vi "APD-counter-synchronized.vi"(0 "ao_to_write":tag="Dev1/ao1", 4 "APD_signal":tag="/Dev1/PFI8", 5 "error in (no error)":errorcluster, 6 "y_start_um":dbl=4.0 format="%.3f", 8 "y_end_um":dbl=6.0 format="%.3f", 10 "Duration_s":dbl=1.0 format="%#_6p", 12 "DAQ sampling rate":dbl=10000.0 format="%#_6p") -> (14 "time tags":u32[](array[numeric])=[1617, 8514, 12274, 20565, 34917, 35402, 37265, 38238, 57954, 68377, 79767, 93435, 95330, 115161, 119575, 126232, 134280, 173482, 175010, 177269, 185202, 187516, 187525, 187814, 188411, 189607, 197427, 217503, 223614, 233596, 240824, 256808, 266059, 270070, 271549, 273666, 274381, 279664, 282850, 287407, 293024, 300860, 320469, 331194, 388082, 391502, 397052, 412341, 413800, 451549, 454051, 488548, 547543, 551076, 552583, 586653, 599650, 613877, 615921, 642961, 646267, 647470, 648566, 683015, 686993, 694317, 710159, 710543, 751020, 763526, 767844, 771220, 794182, 809071, 812953, 822705, 850006, 865624, 875877, 879061, 895901, 900981, 902825, 903577, 906993, 907554, 914434, 916405, 921246, 923738, 936250, 936601, 939722, 948191, 976061, 977403, 979255, 988197, 1004150, 1011377, 1023293, 1025748, 1033762, 1036676, 1037210, 1077098, 1094656, 1098932, 1113325, 1123736, 1123910, 1134400, 1136024, 1143608, 1170409, 1213828, 1232961, 1237449, 1259376, 1267857, 1274171, 1282019, 1286854, 1310462, 1313126, 1315046, 1324275, 1326810, 1332178, 1340368, 1340407, 1343990, 1345221, 1346964, 1364694, 1388750, 1391710, 1403678, 1408248, 1428588, 1444290, 1445629, 1449529, 1452777, 1456715, 1467693, 1479877, 1481248, 1486037, 1497559, 1498462, 1506000, 1507373, 1508422, 1509540, 1510507, 1512549, 1517522, 1522108, 1529163, 1558683, 1564453, 1578897, 1584884, 1589263, 1622523, 1639047, 1640280, 1653969, 1667907, 1686341, 1692400, 1702828, 1706400, 1709526, 1713264, 1716614, 1718721, 1721994, 1735244, 1736688, 1739237, 1762850, 1778098, 1784274, 1786663, 1790948, 1805134, 1810522, 1814629, 1836014, 1840078, 1842022, 1861394, 1878208, 1894207, 1919233, 1923567, 1933515, 1951072, 1951153, 1955923, 1967743, 1970393, 1973969, 1977369, 1978257, 1986658, 1990762, 2017254, 2018231, 2022980, 2036748, 2051136, 2068002, 2077318, 2092650, 2101140, 2112303, 2132887, 2134211, 2164113, 2171564, 2173231, 2188929, 2192828, 2195583, 2196607, 2219129, 2224786, 2229299, 2240229, 2240568, 2248558, 2278572, 2298996, 2305229, 2308700, 2313991, 2345345, 2346179, 2349865, 2350771, 2382508, 2389153, 2390999, 2408371, 2428081, 2433877, 2433926, 2435328, 2437892, 2454139, 2457236, 2475748, 2480449, 2483319, 2492985, 2501361, 2526711, 2532104, 2537449, 2540493, 2545042, 2548591, 2560696, 2566230, 2570890, 2580490, 2600440, 2609949, 2610561, 2611858, 2612448, 2615675, 2635002, 2640843, 2643937, 2658169, 2703087, 2707384, 2712186, 2725379, 2773349, 2775106, 2784948, 2785927, 2786930, 2792713, 2796971, 2814031, 2822352, 2835497, 2835845, 2838919, 2840082, 2841672, 2859967, 2872433, 2879793, 2882072, 2889857, 2897761, 2907259, 2929097, 2963378, 2981447, 2989320, 3002384, 3002385, 3003328, 3011854, 3020261, 3021488, 3029005, 3030028, 3035148, 3059511, 3063096, 3069096, 3077896, 3081773, 3099736, 3146787, 3151070, 3153237, 3159851, 3169791, 3184967, 3190957, 3199514, 3202886, 3205088, 3209452, 3228110, 3235052, 3239233, 3246402, 3247518, 3258710, 3259514, 3276763, 3288042, 3321055, 3321903, 3326046, 3355279, 3358734, 3399824, 3406786, 3423548, 3430377, 3430834, 3432472, 3455758, 3456988, 3465084, 3471831, 3475563, 3497296, 3498536, 3506930, 3509738, 3509998, 3538736, 3538762, 3555497, 3566294, 3571416, 3574354, 3587298, 3594158, 3596294, 3597984, 3609878, 3610183, 3619254, 3623133, 3629713, 3635571, 3641115, 3663964, 3670086, 3679821, 3695717, 3697137, 3706852, 3715146, 3728389, 3766001, 3780817, 3802848, 3808019, 3818393, 3830970, 3843232, 3845469, 3864680, 3872910, 3880489, 3882867, 3896587, 3902984, 3919045, 3927836, 3948484, 3952876, 3958522, 3960194, 3972452, 3977978, 4015413, 4026230, 4031811, 4033763, 4037156, 4073209, 4078826, 4078964, 4088360, 4091171, 4096204, 4103351, 4105273, 4126221, 4130227, 4131168, 4164045, 4166878, 4178284, 4210808, 4214700, 4225379, 4235697, 4239456, 4239652, 4243811, 4244908, 4245750, 4259680, 4266654, 4267090, 4269674, 4277689, 4279478, 4288143, 4289477, 4289528, 4316961, 4318563, 4328159, 4344085, 4350067, 4354935, 4357706, 4365546, 4367346, 4383457, 4388029, 4420363, 4435182, 4436109, 4438820, 4468514, 4478175, 4491660, 4492390, 4497102, 4501457, 4501586, 4512174, 4517070, 4518450, 4536838, 4547886, 4555313, 4556110, 4571596, 4591440, 4602493, 4606762, 4617052, 4644899, 4647553, 4657592, 4672401, 4680982, 4693672, 4696454, 4721246, 4746514, 4748546, 4787883, 4798872, 4811344, 4818805, 4821017, 4828436, 4828492, 4828736, 4841201, 4842107, 4859124, 4865880, 4868886, 4872581, 4879021, 4894944, 4917909, 4922087, 4928487, 4928645, 4964638, 4966510, 4973708, 4983803, 4988440, 4994500, 4998320, 5005289, 5035839, 5039124, 5041040, 5048608, 5052074, 5056335, 5060012, 5074947, 5089912, 5111388, 5118788, 5129501, 5130484, 5156063, 5161939, 5173418, 5176262, 5177784, 5180116, 5217588, 5224915, 5258746, 5268307, 5275408, 5297246, 5309159, 5321253, 5328915, 5330134, 5344478, 5349137, 5365467, 5385955, 5398314, 5404550, 5422605, 5423964, 5431856, 5439427, 5444547, 5459606, 5464748, 5473439, 5480165, 5482909, 5484531, 5508669, 5517179, 5536432, 5552946, 5553034, 5560309, 5565589, 5578409, 5579291, 5596776, 5602314, 5605526, 5612381, 5612652, 5622551, 5629364, 5633164, 5637568, 5647785, 5662593, 5663027, 5678087, 5683696, 5707814, 5708040, 5727142, 5739286, 5743393, 5764846, 5767510, 5778919, 5785074, 5788885, 5790436, 5792182, 5794935, 5815798, 5822258, 5847673, 5849629, 5849702, 5852683, 5853644, 5859227, 5864019, 5866082, 5867143, 5888339, 5896516, 5903365, 5919809, 5927912, 5930228, 5932718, 5936422, 5940913, 5942272, 5953828, 5960268, 5966370, 5967906, 5993952, 5994649, 6000191, 6001891, 6035036, 6038421, 6041090, 6050830, 6052556, 6053826, 6056856, 6057097, 6080835, 6088757, 6091135, 6099057, 6102434, 6114932, 6116858, 6129607, 6141016, 6143043, 6152242, 6156105, 6157624, 6159513, 6161373, 6163582, 6178386, 6187956, 6188493, 6205026, 6233167, 6249963, 6263153, 6264365, 6267125, 6267997, 6270213, 6276638, 6281128, 6286842, 6297236, 6302123, 6307585, 6308029, 6327542, 6344909, 6359615, 6368399, 6369002, 6370874, 6424638, 6439503, 6446102, 6461496, 6463502, 6480104, 6494766, 6496031, 6508645, 6519056, 6523380, 6528804, 6554973, 6556902, 6569896, 6571252, 6581020, 6583224, 6584923, 6599291, 6606595, 6614440, 6624564, 6628476, 6632318, 6637716, 6638169, 6644791, 6650232, 6651619, 6656068, 6667291, 6667510, 6704324, 6706226, 6711263, 6719627, 6724016, 6727619, 6756251, 6765545, 6781244, 6785334, 6798675, 6809716, 6817328, 6820211, 6856900, 6868094, 6899041, 6904923, 6909615, 6919040, 6923653, 6936054, 6939203, 6948855, 6953704, 6956189, 6961686, 6973803, 6976824, 6984715, 7001385, 7014029, 7018130, 7019144, 7023351, 7028702, 7033179, 7039934, 7074129, 7076269, 7077132, 7095149, 7099400, 7104359, 7110045, 7115025, 7126495, 7135263, 7158151, 7162036, 7187178, 7189383, 7194225, 7208639, 7208746, 7213943, 7282317, 7299353, 7301721, 7314437, 7316458, 7326789, 7334609, 7337898, 7339472, 7344845, 7346255, 7349370, 7356432, 7366135, 7374208, 7376719, 7380782, 7388813, 7388943, 7397243, 7401920, 7408246, 7416961, 7434816, 7435896, 7439219, 7454399, 7455070, 7459639, 7474225, 7490642, 7491990, 7502524, 7506416, 7511657, 7511671, 7514649, 7519099, 7530651, 7536651, 7549344, 7562326, 7563224, 7564770, 7569785, 7577790, 7583357, 7586769, 7589907, 7592271, 7602685, 7615016, 7621713, 7627357, 7659690, 7661778, 7669294, 7669581, 7681622, 7705966, 7711336, 7713905, 7715976, 7725547, 7737879, 7748149, 7754644, 7757162, 7758005, 7760640, 7774067, 7782750, 7800584, 7806004, 7807595, 7810954, 7812385, 7831951, 7844263, 7852555, 7859270, 7875341, 7891990, 7893385, 7909423, 7917565, 7922227, 7970722, 7973979, 7976651, 7986173, 7988731, 7996540, 7997442, 8002024, 8005784, 8008548, 8015237, 8016979, 8018636, 8031638, 8036817, 8051972, 8052911, 8061175, 8063984, 8071339, 8075799, 8080806, 8082777, 8092643, 8095235, 8101005, 8103243, 8103501, 8105684, 8108064, 8118580, 8130143, 8131594, 8139319, 8142296, 8147224, 8150515, 8157836, 8162474, 8167935, 8169793, 8173237, 8174026, 8174599, 8190819, 8198129, 8216513, 8218408, 8227556, 8230675, 8232058, 8232376, 8237816, 8252618, 8264563, 8276111, 8287066, 8309355, 8310996, 8316353, 8330239, 8332140, 8346844, 8354814, 8379426, 8400413, 8415506, 8417231, 8429309, 8429562, 8448711, 8453931, 8465139, 8468917, 8476213, 8491690, 8507968, 8512199, 8521587, 8525347, 8530588, 8532568, 8533136, 8533606, 8535767, 8542964, 8551744, 8557349, 8568057, 8579623, 8591329, 8630869, 8631263, 8641524, 8641540, 8645573, 8657240, 8659153, 8661211, 8670372, 8671613, 8688464, 8700013, 8705979, 8711129, 8716432, 8727138, 8732652, 8754294, 8760296, 8773752, 8775389, 8792686, 8798218, 8806915, 8806957, 8808256, 8808423, 8810238, 8811551, 8815337, 8815338, 8823424, 8824807, 8831585, 8833635, 8842125, 8849130, 8855007, 8861026, 8862986, 8867363, 8882422, 8902876, 8905207, 8906718, 8911015, 8930178, 8932604, 8943618, 8954223, 8958968, 8959609, 8980355, 8980858, 8985305, 8998408, 9009003, 9036042, 9040401, 9044806, 9047366, 9052151, 9067578, 9068225, 9127447, 9145363, 9146347, 9149805, 9157603, 9162213, 9166615, 9170985, 9184377, 9192907, 9198452, 9201877, 9204403, 9212852, 9214432, 9223940, 9224233, 9228419, 9232814, 9238431, 9239957, 9249919, 9255933, 9262012, 9268098, 9279058, 9279456, 9287255, 9295881, 9296488, 9304065, 9316119, 9343190, 9357714, 9364199, 9365191, 9369210, 9378347, 9387386, 9405033, 9435254, 9437668, 9437972, 9438398, 9440121, 9440983, 9449780, 9455423, 9456955, 9463983, 9495248, 9504104, 9554094, 9573156, 9580807, 9582784, 9591248, 9592954, 9597285, 9605408, 9605979, 9606407, 9616770, 9632422, 9635038, 9647403, 9684806, 9696212, 9722896, 9725217, 9729213, 9740910, 9752284, 9774418, 9786059, 9787440, 9788436, 9795933, 9804987, 9809372, 9812795, 9822094, 9827265, 9833549, 9837013, 9837305, 9840632, 9840891, 9849124, 9856510, 9870947, 9890659, 9892186, 9898537, 9912117, 9914470, 9921183, 9942452, 9948337, 9957854, 9959132, 9964622, 9976656, 9987644, 9999037, 10001684, 10004443, 10025300], 15 "counts":i32=1118, 16 "clock cycles":i32=10000000, 19 "error out":errorcluster)   [LabVIEW 2018]
uses:
  <vilib>/Analysis/1siggen.llb/Ramp Pattern by Samples.vi
  GLOBAL_VAR.vi
  <vilib>/Analysis/NI_AALBase.lvlib
panel:
  out "signal_to_write":waveform(dbl)(graph)={"t0"=timestamp(0 s since 1904-01-01), "dt"=0.0001, "Y"=array[10000 elements]}
  out "#daq samples":i32=10000
  # "Analog Output is a linear ramp"
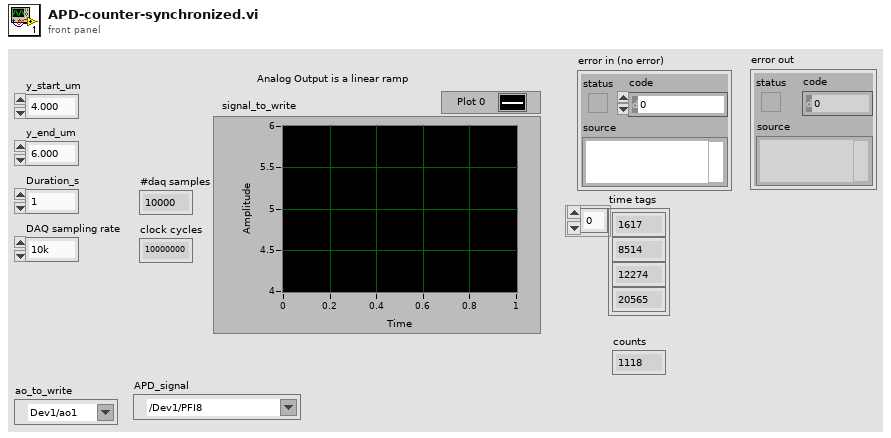
[diagram p1: front panel]
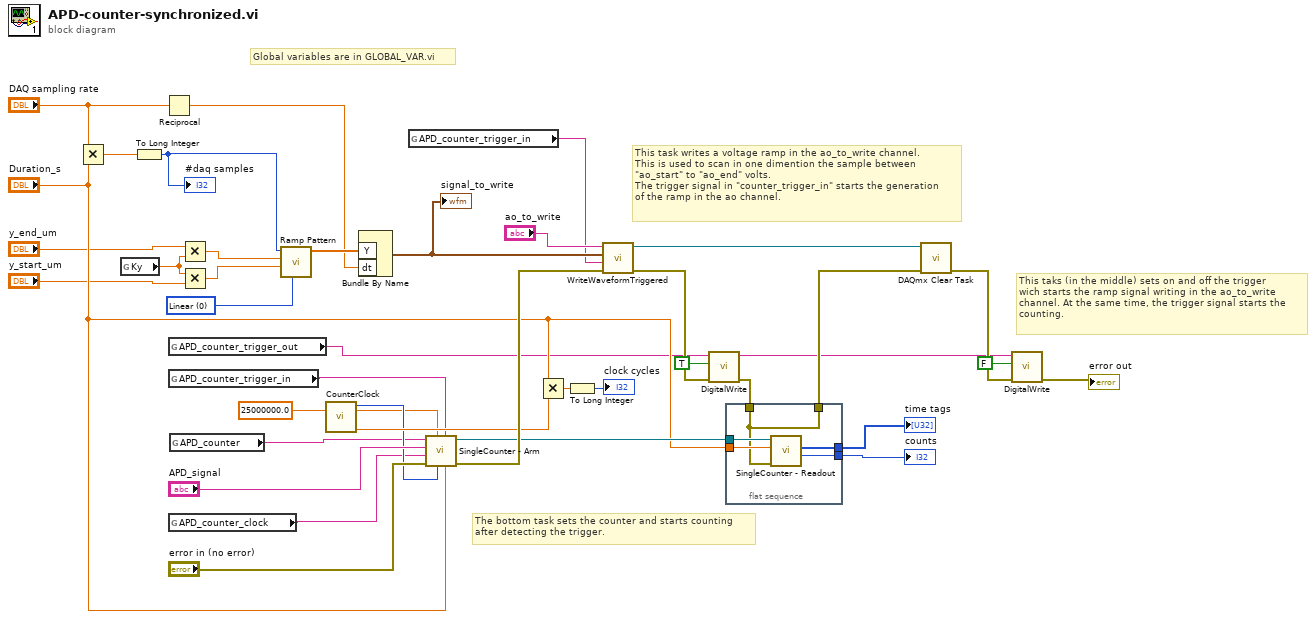
[diagram p0: block diagram]
diagram:
  w25 = u16 0 items=["Linear", "Logarithmic"] ("type")
  # "Global variables are in GLOBAL_VAR.vi"
  # "The bottom task sets the counter and starts counting\nafter detecting the trigger."
  # "This taks (in the middle) sets on and off the trigger\nwich starts the ramp signal writing in the ao_to_write\nchannel. At the same time, the trigger signal starts the \ncounting."
  # "This task writes a voltage ramp in the ao_to_write channel.\nThis is used to scan in one dimention the sample between \n\"ao_start\" to \"ao_end\" volts.\nThe trigger signal in \"counter_trigger_in\" starts the generation\nof the ramp in the ao channel."
  n1 = Multiply(x="DAQ sampling rate", y="Duration_s") -> (x*y=w26:dbl)
  n2 = global read "GLOBAL_VAR.vi" "Ky"() -> (w1:dbl)
  n3 = To Long Integer(number=w26) -> (32bit integer=w21:i32)
  "#daq samples" <- w21
  n4 = Reciprocal(x="DAQ sampling rate") -> (1/x=w22:dbl)
  n5 = global read "GLOBAL_VAR.vi" "APD_counter_trigger_out"() -> (w9:tag)
  n6 = global read "GLOBAL_VAR.vi" "APD_counter_trigger_in"() -> (w8:tag)
  n7 = global read "GLOBAL_VAR.vi" "APD_counter_clock"() -> (w6:tag)
  n8 = global read "GLOBAL_VAR.vi" "APD_counter"() -> (w7:tag)
  n9 = Multiply(x="y_end_um", y=w1) -> (x*y=w5:dbl)
  n10 = Multiply(x=w1, y="y_start_um") -> (x*y=w4:dbl)
  n11 = call-poly <vilib>:"Ramp Pattern.vi"("type"=w25, "start"=w4, "end"=w5, "samples"=w21) -> ("Ramp Pattern"=w23:dbl[])  [unwired: 6 in, 1 out]
  n12 = call "CounterClock.vi"() -> ("Counter clock rate divided by prescaler"=w14:dbl, "CI.Prescaler"=w13:u32)  [unwired: 8 in, 2 out]
  n13 = Bundle By Name("Y"=w23, "dt"=w22) -> (w20:waveform(dbl))  [unwired: 1 in]
  "signal_to_write" <- w20
  n14 = global read "GLOBAL_VAR.vi" "APD_counter_trigger_in"() -> (w10:tag)
  n15 = call "SingleCounter - Arm.vi"("Duration"="Duration_s", "Trigger Source"=w8, "CI.Prescaler"=w13, "Sampling Rate"=25000000.0, "Error In"="error in (no error)", "Clock Source"=w6, "External Timing Source"="APD_signal", "counter"=w7) -> ("error out"=w32:errorcluster, "task out"=w31:refnum<k21>)  [unwired: 2 in]
  n16 = Multiply(x="Duration_s", y=w14) -> (x*y=w17:dbl)
  n17 = To Long Integer(number=w17) -> (32bit integer=→"clock cycles":i32)
  n18 = call "WriteWaveformTriggered.vi"("error in (no error)"=w32, "Trigger source"=w10, "waveform in"=w20, "physical channel"="ao_to_write") -> ("error out"=w27:errorcluster, "task out"=w37:refnum<k21>)  [unwired: 6 in]
  n19 = call "DigitalWrite.vi"("error in (no error)"=w27, "on/off"=TRUE ("data"), "lines"=w9) -> ("error out"=w16:errorcluster)  [unwired: 8 in]
  n20 = flat-sequence {
    tunnel: w31 -> [w43]
    tunnel: [w42] -> w30
    tunnel: [w41] -> w29
    tunnel: "Duration_s" -> [w40]
    tunnel: w16 -> [w39]
    tunnel: [w39] -> w15
    frame #0 {
      n21 = call "SingleCounter - Readout.vi"("Error In"=w39, "seconds to wait"=w40, "task in"=w43) -> ("counts"=w41:i32, "time tags"=w42:u32[])  [unwired: 6 in, 1 out]
    }
  }
  n22 = call <vilib>:"DAQmx Clear Task.vi"("task in"=w37, "error in"=w15) -> ("error out"=w36:errorcluster)  [unwired: 13 in]
  n23 = call "DigitalWrite.vi"("error in (no error)"=w36, "on/off"=FALSE ("data"), "lines"=w9) -> ("error out"=→"error out":errorcluster)  [unwired: 8 in]
  "time tags" <- w30
  "counts" <- w29
